vi "LvMPDC_CMD_Playlist_clear.vi"(6 "timeout_ms":i32=3000, 8 "error in (no error)":errorcluster, 9 "ReadBytes":i32=1024, 11 "Connect ID":refnum<k5>) -> (0 "error out":errorcluster, 3 "Connect ID out":refnum<k5>)   [LabVIEW 2012]
panel:
  in  "pos":i32=-1
  # "LvMPDC:: CMD clear (clear Playlist)"
  # "-1 は番号指定無し"
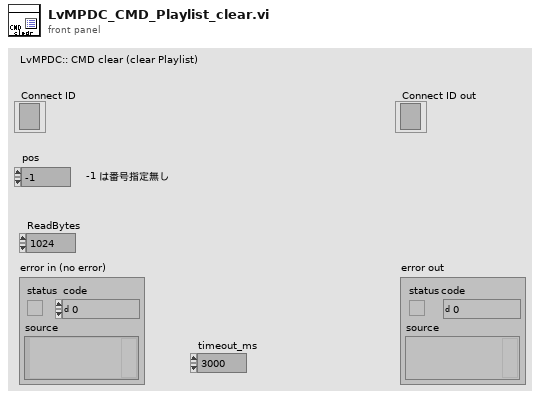
[diagram p1: front panel]
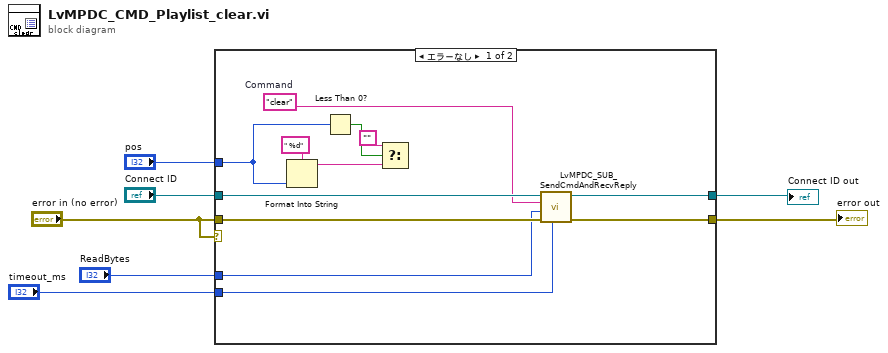
[diagram p0: block diagram]
diagram:
  n1 = case shown="エラーなし" "error in (no error)" {
    tunnel: "Connect ID" -> [w17 w21]
    tunnel: "error in (no error)" -> [w19 w20]
    tunnel: [w16 w21] -> w6
    tunnel: [w18 w20] -> w5
    tunnel: "timeout_ms" -> [w14 _]
    tunnel: "ReadBytes" -> [w15 _]
    tunnel: "pos" -> [w12 _]
    frame No Error {
      w8 = "clear"  # Command
      n2 = Format Into String(format string=" %d" ("形式文字列"), w12) -> (resulting string=w9:string)  [unwired: 2 in, 1 out]
      n3 = Less Than 0?(x=w12) -> (x < 0?=w11:bool)
      n4 = Select(t="", s=w11, f=w9) -> ()  [unwired: 1 out]
      n5 = call "LvMPDC_SUB_SendCmdAndRecvReply.vi"("timeout_ms"=w14, "error in (no error)"=w19, "ReadBytes"=w15, "Command"=w8, "Connect ID"=w17) -> ("error out"=w18:errorcluster, "Connect ID out"=w16:refnum<k5>)  [unwired: 4 in, 1 out]
    }
    frame Error {
    }
  }
  "Connect ID out" <- w6
  "error out" <- w5
